vi "Assign UDP Port to Aircraft.vi"(8 "error out":errorcluster, 11 "UDP Port Ref":refnum<k16>) -> (0 "error out":errorcluster, 1 "Aircraft ID":u8, 2 "Message Complete":bool, 3 "UDP Ref Out":refnum<k16>, 4 "IP Address":string)   [LabVIEW 2014]
uses:
  Application Support/Stop Button/SubVI/Get Stop Button Status.vi
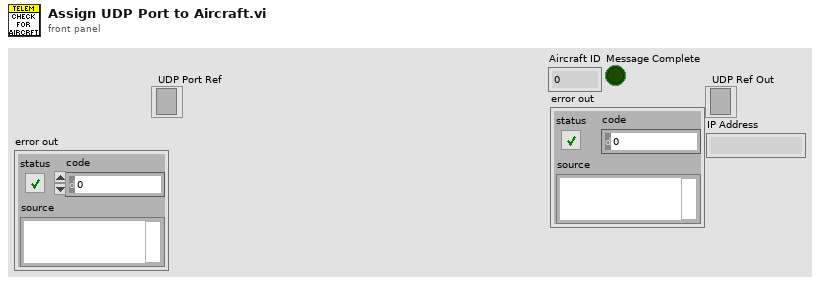
[diagram p1: front panel]
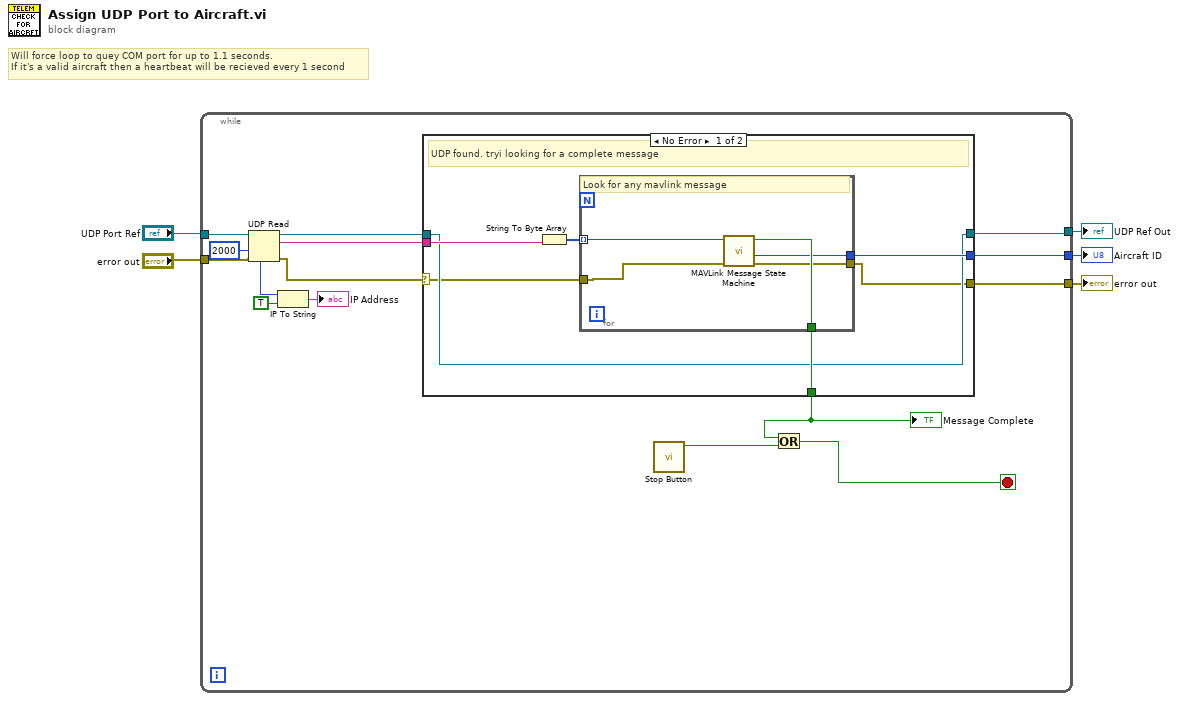
[diagram p0: block diagram]
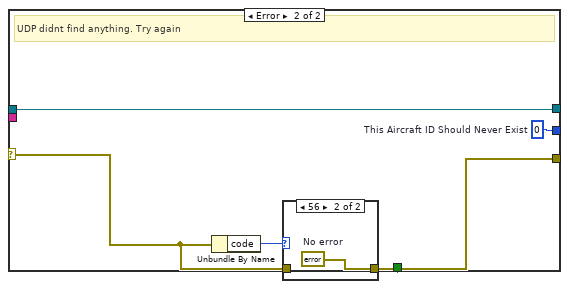
[diagram p2: hidden frame]
diagram:
  # "Will force loop to quey COM port for up to 1.1 seconds.\nIf it's a valid aircraft then a heartbeat will be recieved every 1 second"
  n1 = while {
    tunnel: "UDP Port Ref" -> [w14]
    tunnel: "error out" -> [w13]
    tunnel: [w20] -> w4
    tunnel: [w19] -> w3
    tunnel: [w18] -> w1
    stop <- w16 stop-if-true
    n2 = UDP Read(connection ID=w14, timeout ms (25000)=2000, 8:w13) -> (data out=w10:string, error out=w11:errorcluster, 3:w12:refnum<k16>, 6:w8:u32)  [unwired: 2 out]
    n3 = IP To String(1:TRUE ("dot notation? (F)"), 2:w8) -> (0:→"IP Address":string)
    n4 = case shown="No Error" w11 {
      selector: w11 -> [w22 w33]
      tunnel: w12 -> [w23 w36]
      tunnel: [w26 w38] -> w17
      tunnel: [w25 w37] -> w20
      tunnel: [w21 w34] -> w19
      tunnel: [w23 w36] -> w18
      tunnel: w10 -> [w24 _]
      frame No Error {
        # "UDP found. tryi looking for a complete message"
        n5 = String To Byte Array(string=w24) -> (unsigned byte array=w27:u8[])
        n6 = for {
          tunnel: w27 -> [w32] mode=indexing
          tunnel: [w31] -> w26
          tunnel: [w30] -> w25
          tunnel: w22 -> [w29]
          tunnel: [w28] -> w21
          # "Look for any mavlink message"
          n7 = call "MAVLink Message State Machine.vi"("Error In"=w29, "Incoming Bytes"=w32) -> ("Error Out"=w28:errorcluster, "Aircraft ID"=w30:u8, "Message Complete"=w31:bool)  [unwired: 6 in, 1 out]
        }
      }
      frame Error {
        w37 = u8 0  # This Aircraft ID Should Never Exist
        w38 = FALSE  # Message Complete? Try again
        # "UDP didnt find anything. Try again"
        n8 = Unbundle By Name(w33) -> ("code"=w35:i32)
        n9 = case shown="56" w35 {
          tunnel: w33 -> [w39 _]
          tunnel: [w39 w40] -> w34
          frame Default {
          }
          frame 56 {
            w40 = errorcluster {"status"=FALSE, "code"=0, "source"=""}  # No error
          }
        }
      }
    }
    "Message Complete" <- w17
    n10 = call-poly "Stop Button.vi"() -> ("Stop ButtonOut"=w15:bool)  [unwired: 10 in, 1 out]
    n11 = Or(x=w17, y=w15) -> (x .or. y?=w16:bool)
  }
  "Aircraft ID" <- w4
  "error out" <- w3
  "UDP Ref Out" <- w1
